vi "initEncoders.vi"(8 "error in (no error)":errorcluster, 9 "Left Encoder":string="LeftEncoder", 10 "Right Encoder":string="RightEncoder") -> (0 "error out":errorcluster)   [LabVIEW 2013]
uses:
  <vilib>/Rock Robotics/SystemInterfaces/DIO/FPGA_DIOChannel.ctl
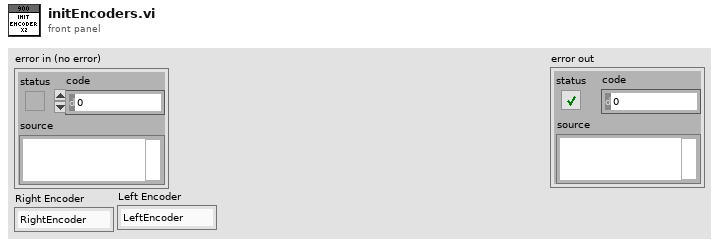
[diagram p1: front panel]
types:
  T1 = typedef "FPGA_DIOChannel.ctl" = enum8{"DIO 1", "DIO 2", "DIO 3", "DIO 4", "DIO 5", "DIO 6", "DIO 7", "DIO 8", "DIO 9", "DIO 10", "DIO 11", "DIO 12", "DIO 13", "DIO 14", "Invalid"}
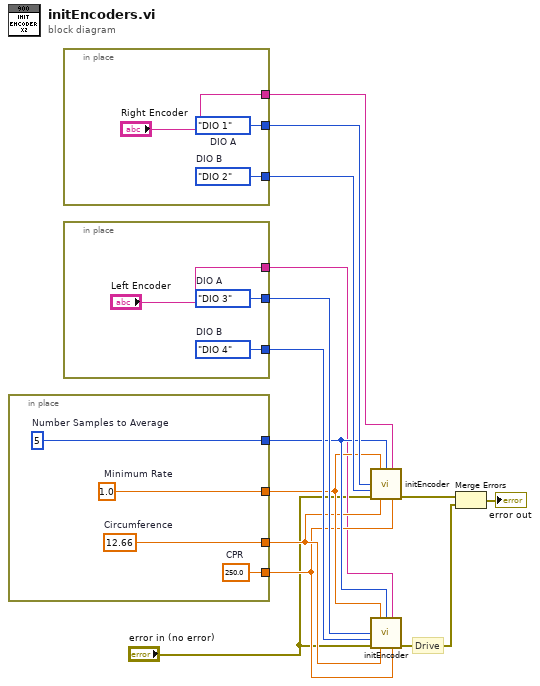
[diagram p0: block diagram]
diagram:
  # "Drive"
  n1 = in-place {
    in-place-border: [w18] -> w9
    in-place-border: [w17] -> w8
    in-place-border: [w16] -> w7
    in-place-border: [w15] -> w6
    w15 = 250.0  # CPR
    w16 = 12.66  # Circumference
    w17 = 1.0  # Minimum Rate
    w18 = u8 5  # Number Samples to Average
  }
  n2 = in-place {
    in-place-border: [w21] -> w14
    in-place-border: [w20] -> w13
    in-place-border: ["Right Encoder"] -> w10
    w20 = FPGA_DIOChannel."DIO 2"  # DIO B
    w21 = FPGA_DIOChannel."DIO 1"  # DIO A
  }
  n3 = in-place {
    in-place-border: [w24] -> w12
    in-place-border: [w23] -> w11
    in-place-border: ["Left Encoder"] -> w5
    w23 = FPGA_DIOChannel."DIO 4"  # DIO B
    w24 = FPGA_DIOChannel."DIO 3"  # DIO A
  }
  n4 = call "initEncoder.vi"("Minimum Rate"=w8, "Number Samples to Average"=w9, "refnum name"=w10, "DIO A"=w14, "DIO B"=w13, "error in (no error)"="error in (no error)", "Circumference"=w7, "CPR"=w6) -> ("error out"=w4:errorcluster)  [unwired: 7 in]
  n5 = call "initEncoder.vi"("Minimum Rate"=w8, "Number Samples to Average"=w9, "refnum name"=w5, "DIO A"=w12, "DIO B"=w11, "error in (no error)"="error in (no error)", "Circumference"=w7, "CPR"=w6) -> ("error out"=w3:errorcluster)  [unwired: 7 in]
  n6 = Merge Errors(w4, w3) -> (→"error out":errorcluster)
